vi "Close.vi"(5 "error in (no error)":errorcluster) -> (19 "error out":errorcluster)   [LabVIEW 2017, in "G#RemoteProxy.lvclass"]
doc: "Closes proxy objects."
uses:
  <vilib>/addons/_AddQ/G#Debugger/G#RemoteProxy/G#RemoteProxy.lvclass
  C:/Program Files (x86)/National Instruments/LabVIEW 2017/vi.lib/addons/_AddQ/G#Object/G#Object.lvclass
  <vilib>/addons/_AddQ/G#Object/G#Object.lvclass
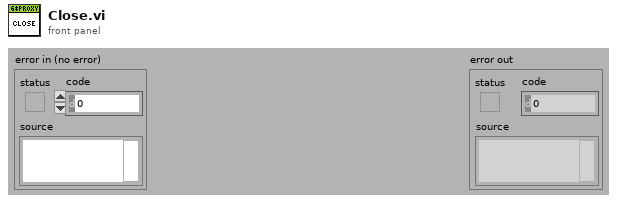
[diagram p1: front panel]
types:
  T1 = typedef "G#RemoteProxy.lvclass/ClassAttributesRef.ctl" = refnum<data-value>
  T2 = typedef "G#RemoteProxy.lvclass/ClassAttributesProxy.ctl" = cluster{"NoActiveProject":bool, "FullClassNames":string[], "FullClassPaths":path[], "RemoteRefs":refnum<class "G#Object.lvclass">[], "ProxyRefs":refnum<class "G#RemoteProxy.lvclass">[], "RemoteClassName":string[], "ProxyClassRefs":refnum<class "G#RemoteProxy.lvclass">[]}
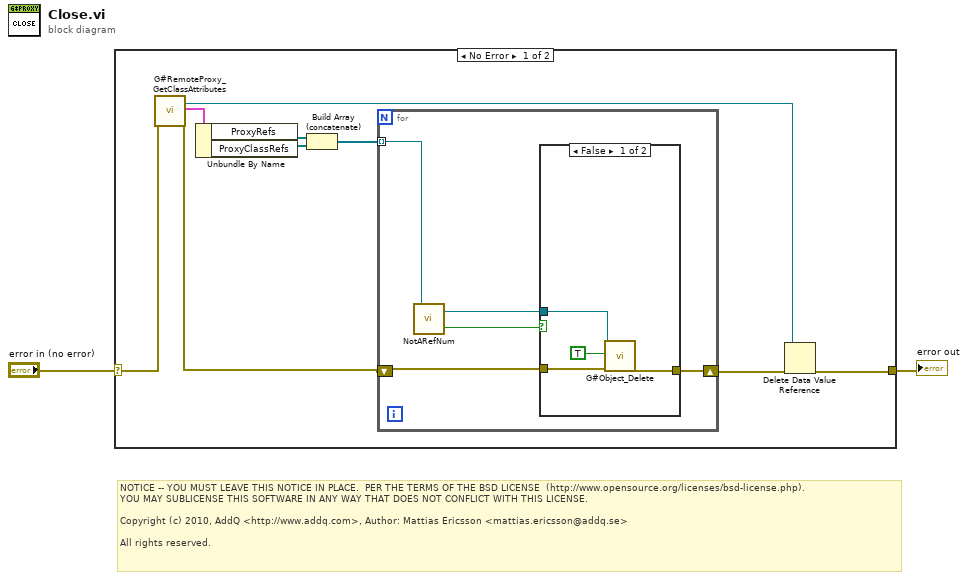
[diagram p0: block diagram]
diagram:
  # "NOTICE -- YOU MUST LEAVE THIS NOTICE IN PLACE.  PER THE TERMS OF THE BSD LICENSE  (http://www.opensource.org/licenses/bsd-license.php).\nYOU MAY SUBLICENSE THIS SOFTWARE IN ANY WAY THAT DOES NOT CONFLICT WITH THIS LICENSE.\n\nCopyright (c) 2010, AddQ <http://www.addq.com>, Author: Mattias Ericsson <mattias.ericsson@addq.se>\n\nAll rights reserved."
  n1 = case shown="No Error" "error in (no error)" {
    selector: "error in (no error)" -> [w11 w22]
    tunnel: [w4 w22] -> w1
    frame No Error {
      n2 = call <vilib>:"G#RemoteProxy_GetClassAttributes.vi"("error in (no error)"=w11) -> ("class attributes ref"=w3:T1, "class attributes"=w10:T2, "error out"=w9:errorcluster)  [unwired: 15 in, 1 out]
      n3 = Unbundle By Name(w10) -> ("ProxyRefs"=w7:refnum<class "G#RemoteProxy.lvclass">[], "ProxyClassRefs"=w8:refnum<class "G#RemoteProxy.lvclass">[])
      n4 = Build Array (concatenate)(w7, w8) -> (w6:refnum<class "G#RemoteProxy.lvclass">[])
      n5 = for {
        shift-right: [w16] -> w5
        shift-left: w9 -> [w15]
        tunnel: w6 -> [w14] mode=indexing
        n6 = call-dynamic "NotARefNum.vi"("reference in"=w14) -> ("not a refnum?"=w12:bool, "reference out"=w13:refnum<class "G#RemoteProxy.lvclass">)  [unwired: 1 in]
        n7 = case shown="False" w12 {
          tunnel: [w20 w21] -> w16
          tunnel: w15 -> [w19 w21]
          tunnel: w13 -> [w18 _]
          frame False {
            n8 = call <vilib>:"G#Object_Delete.vi"("reference in"=w18, "force delete? (F)"=TRUE, "error in (no error)"=w19) -> ("error out"=w20:errorcluster)  [unwired: 15 in, 1 out]
          }
          frame True {
          }
        }
      }
      n9 = Delete Data Value Reference(data value reference=w3, error in=w5) -> (error out=w4:errorcluster)  [unwired: 1 out]
    }
    frame Error {
    }
  }
  "error out" <- w1
